vi "Monitor.vi"() -> ()   [LabVIEW 2018]
uses:
  <vilib>/Enthought/Python Integration Toolkit/api/Console Visibility.ctl
  Global Variables.vi
  <vilib>/Utility/file.llb/Read Delimited Spreadsheet (string).vi
  <vilib>/Enthought/Python Integration Toolkit/api/Unpack Bool.vi
  <vilib>/Enthought/Python Integration Toolkit/Python Integration Toolkit.lvlib
panel:
  out "Last Event Recording":string="10:59:18 AM"
  out "Sensors Info":T1(array[cluster])=[{"Label.Text"="", "Panel Ref Out"=refnum, TRUE}]
  out "Instruments":T2(array[cluster])=[{"Name"="Chassis_Sensors.vi", "vi reference"=refnum, "Running?"=TRUE}]
  in  "Add Custom Event":bool
  in  "Custom Event Str":string
  in  "Ring":u16(ring) items=["Proj_VaporTubes", "Proj_H2DT", "Proj_H2DT"]
  in  "Global File Information":T3={"Ring"=0, "SubFolder"="Temp Dependence", "Filename (Meas. Description)"="300C", "Measurement index"=5} {"Ring" items=["Proj_VaporTubes", "Proj_H2DT", "Proj_H2DT"]}
  out "File Size (Mb)":dbl[](array[numeric])
  in  "stop":bool
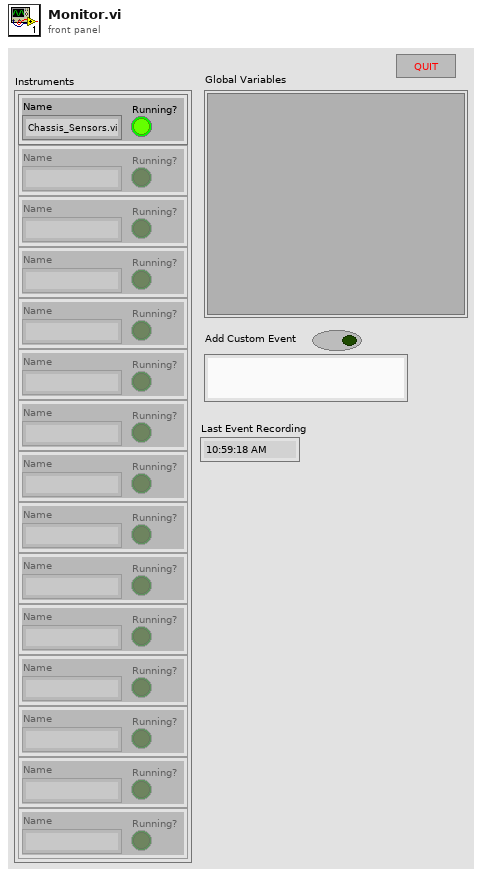
[diagram p1: front panel]
types:
  T1 = cluster{"Label.Text":string, "Panel Ref Out":refnum<vi>, bool}[]
  T2 = cluster{"Name":string, "vi reference":refnum<vi>, "Running?":bool}[]
  T3 = cluster{"Ring":u16, "SubFolder":string, "Filename (Meas. Description)":string, "Measurement index":i32}
  T4 = typedef "Python Integration Toolkit.lvlib/Console Visibility.ctl" = enum16{"Show Console", "Show Console While Running", "Hide Console"}
  T5 = enum32{"Bad", "Idle", "Run top level", "Running"}
  T6 = typedef "Python Integration Toolkit.lvlib/Session ID.ctl" = u64
  T7 = cluster{"Name":string, "vi reference":refnum<vi>, bool}
  T8 = cluster{"Name":string, "vi reference":refnum<vi>, bool}[]
  T9 = typedef "Python Integration Toolkit.lvlib/Python Objects.ctl" = variant
  T10 = cluster{"Project":u16, "SubFolder":string, "Filename (Meas. Description)":string, "Measurement index":i32}
  T11 = cluster{"Project 2":u16, "SubFolder 2":string, "Meas. Description 2":string, "Measurement number 2":i32}
  T12 = cluster{"Label.Text":bool, "Panel Ref Out":bool, bool}[]
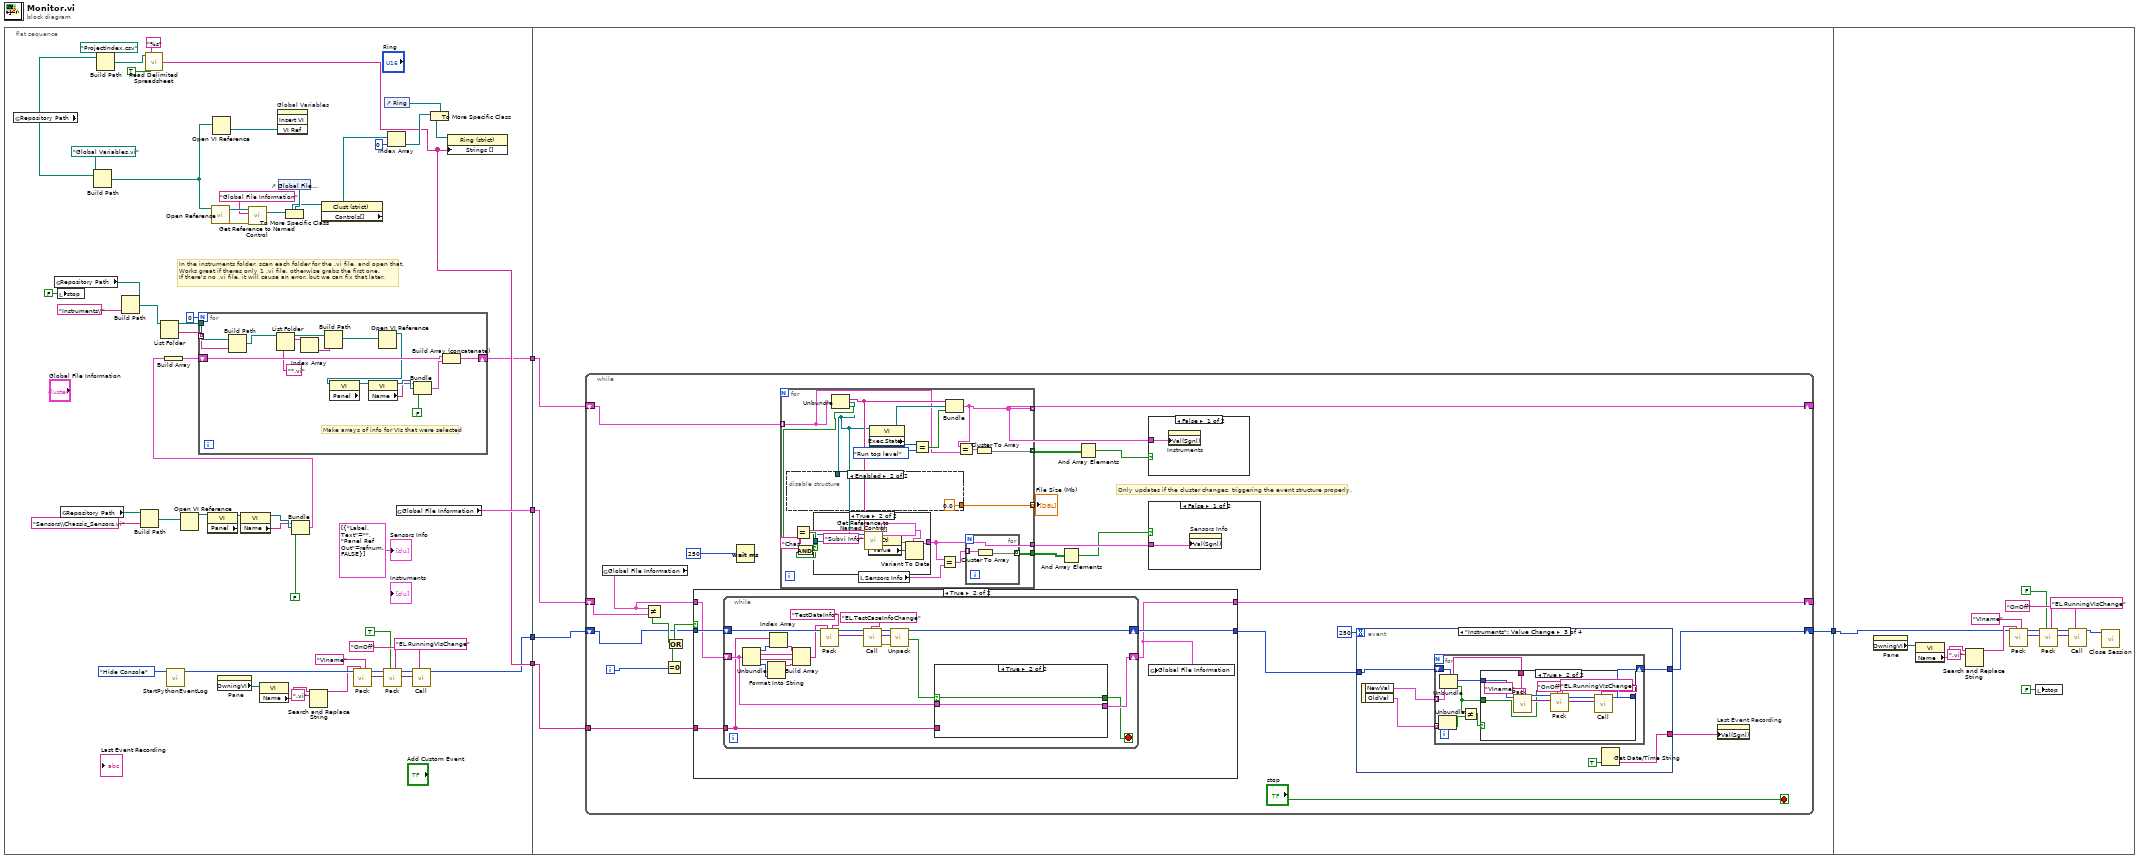
[diagram p0: block diagram]
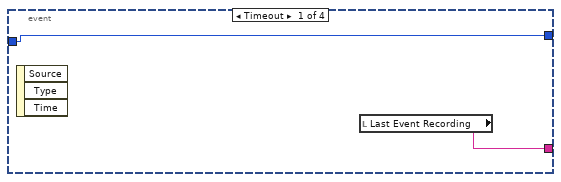
[diagram p4: hidden frame]
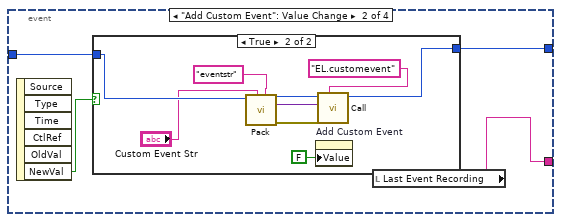
[diagram p5: hidden frame]
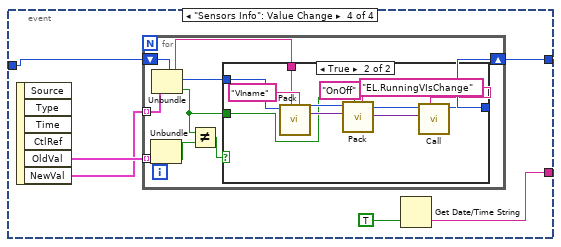
[diagram p8: hidden frame]
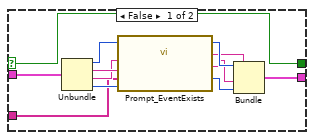
[diagram p11: hidden frame]
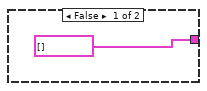
[diagram p12: hidden frame]
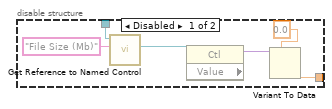
[diagram p13: hidden frame]
diagram:
  n1 = flat-sequence {
    tunnel: [w28] -> w5
    tunnel: [w41] -> w4
    tunnel: [w18] -> w2
    tunnel: [w38] -> w1
    tunnel: w5 -> [w78]
    tunnel: w4 -> [w81]
    tunnel: [w80] -> w3
    tunnel: w2 -> [w79]
    tunnel: w1 -> [w77]
    tunnel: w3 -> [w255]
    frame #0 {
      # "In the instruments folder, scan each folder for the .vi file, and open that.\nWorks great if theres only 1 .vi file, otherwise grabs the first one.\nIf there's no .vi file, it will cause an error, but we can fix that later."
      n2 = global read "Global Variables.vi" "Repository Path"() -> (w39:path)
      n3 = global read "Global Variables.vi" "Repository Path"() -> (w23:path)
      n4 = local write "stop"(FALSE ("stop")) -> ()
      n5 = global read "Global Variables.vi" "Repository Path"() -> (w17:path)
      n6 = Build Path(base path=w39, name or relative path=path "Global Variables.vi" ("vi path")) -> (appended path=w54:path)
      n7 = Build Path(base path=w39, name or relative path=path "ProjectIndex.csv" ("vi path")) -> (appended path=w42:path)
      n8 = Build Path(base path=w23, name or relative path="Instruments\\") -> (appended path=w21:path)
      n9 = Build Path(base path=w17, name or relative path="Sensors\\Chassis_Sensors.vi") -> (appended path=w15:path)
      n10 = call-poly <vilib>:"Read Delimited Spreadsheet.vi"("file path (dialog if empty)"=w42, "format (%s)"="%s", "transpose? (F)"=TRUE) -> ("first row"=w38:string[])  [unwired: 7 in, 5 out]
      n11 = List Folder(path=w21) -> (path out=w19:path, folder names=w20:string[])  [unwired: 3 in, 2 out]
      n12 = call "StartPythonEventLog.vi"("Console Visibility"=Console_Visibility."Hide Console") -> ("Session ID out"=w29:T6)  [unwired: 10 in]
      n13 = Open VI Reference(vi path=w15) -> (vi reference=w10:refnum<vi>)  [unwired: 5 in, 1 out]
      n14 = property class="VI" props=["Panel"](reference=w10) -> (reference out=w14:refnum<vi>)  [unwired: 1 in, 2 out]
      n15 = call "Open Reference.vi"("vi path"=w54) -> ("error out"=w55:errorcluster, "Front Panel Reference"=w56:refnum<vi>)  [unwired: 5 in]
      n16 = Open VI Reference(vi path=w54) -> (vi reference=w60:refnum<vi>)  [unwired: 5 in, 1 out]
      n17 = property on="Pane" class="Pane"() -> ("OwningVI"=w27:refnum<vi>)  [unwired: 2 in, 2 out]
      n18 = property class="VI"(reference=w14) -> (reference out=w13:refnum<vi>, "Name"=w11:string)  [unwired: 1 in, 1 out]
      n19 = call "Get Reference to Named Control.vi"("error in (no error)"=w55, "Control Name"="Global File Information", "Front Panel Ref"=w56) -> ("Ctl Refnum"=w52:refnum<vi>)  [unwired: 6 in, 2 out]
      n20 = property class="VI"(reference=w27) -> ("Name"=w26:string)  [unwired: 1 in, 2 out]
      n21 = invoke on="Global Variables" class="SubPnl" method="Insert VI"("VI Ref"=w60) -> ()  [unwired: 3 in, 4 out]
      n22 = control-ref of="Global File Information"() -> (w51:refnum<vi>)
      n23 = To More Specific Class(target class=w51, reference=w52) -> (specific class reference=w50:refnum<vi>)  [unwired: 1 in, 1 out]
      n24 = Bundle("Name"=w11, "vi reference"=w13, FALSE) -> (w9:T7)  [unwired: 1 in]
      n25 = Build Array(w9) -> (w8:T8)
      n26 = for {
        N: 0 -> [_]
        shift-right: [w75] -> w18
        shift-left: w8 -> [w76]
        tunnel: w19 -> [w69]
        tunnel: w20 -> [w68] mode=indexing
        # "Make arrays of info for VIs that were selected"
        n27 = Build Path(base path=w69, name or relative path=w68) -> (appended path=w63:path)
        n28 = List Folder(path=w63, pattern="*.vi") -> (path out=w62:path, filenames=w66:string[])  [unwired: 2 in, 2 out]
        n29 = Index Array(array=w66) -> (element=w65:string)  [unwired: 1 in]
        n30 = Build Path(base path=w62, name or relative path=w65) -> (appended path=w67:path)
        n31 = Open VI Reference(vi path=w67) -> (vi reference=w73:refnum<vi>)  [unwired: 5 in, 1 out]
        n32 = property class="VI" props=["Panel"](reference=w73) -> (reference out=w72:refnum<vi>)  [unwired: 1 in, 2 out]
        n33 = property class="VI"(reference=w72) -> (reference out=w71:refnum<vi>, "Name"=w61:string)  [unwired: 1 in, 1 out]
        n34 = Bundle("Name"=w61, "vi reference"=w71, FALSE) -> (w74:T7)  [unwired: 1 in]
        n35 = Build Array (concatenate)(w76, w74) -> (w75:T8)
      }
      n36 = Search and Replace String(input string=w26, search string=".vi") -> (result string=w24:string)  [unwired: 6 in, 3 out]
      n37 = property class="Clust (strict)"(reference=w50) -> ("Controls[]"=w49:refnum<vi>[])  [unwired: 1 in, 2 out]
      n38 = call <vilib>:"Pack.vi"("Keyword Name"="VIname", "Argument"=w24, "Session ID"=w29) -> ("Python Object References Out"=w33:T9, "Session ID out"=w35:T6)  [unwired: 6 in, 1 out]
      n39 = call <vilib>:"Pack.vi"("Keyword Name"="OnOff", "Argument"=TRUE, "Python Object References In"=w33, "Session ID"=w35) -> ("Python Object References Out"=w32:T9, "Session ID out"=w34:T6)  [unwired: 5 in, 1 out]
      n40 = control-ref of="Ring"() -> (w47:refnum<vi>)
      n41 = Index Array(array=w49, index=0) -> (element=w46:refnum<vi>)
      n42 = global read "Global Variables.vi" "Global File Information"() -> (w41:T10)
      n43 = call <vilib>:"Call.vi"("Function or Method Name"="EL.RunningVIsChange", "Python Object References In"=w32, "Session ID"=w34) -> ("Session ID out"=w28:T6)  [unwired: 6 in, 2 out]
      n44 = To More Specific Class(target class=w47, reference=w46) -> (specific class reference=w45:refnum<vi>)  [unwired: 1 in, 1 out]
      n45 = property class="Ring (strict)"(reference=w45, "Strings []"=w38) -> ()  [unwired: 1 in, 2 out]
      "Sensors Info" <- T1 [{"Label.Text"="", "Panel Ref Out"=refnum, FALSE}] ("Sensors Info")
    }
    frame #1 {
      n46 = while {
        shift-right: [w96] -> _
        shift-left: w81 -> [w97]
        shift-right: [w88] -> _
        shift-left: w79 -> [w87]
        shift-right: [w91] -> w80
        shift-left: w78 -> [w94]
        tunnel: w77 -> [w93]
        i -> [w100]
        stop <- "stop" stop-if-true
        # "Only updates if the cluster changes, triggering the event structure properly."
        n47 = global read "Global Variables.vi" "Global File Information"() -> (w99:T10)
        n48 = Not Equal?(x=w99, y=w97) -> (x != y?=w102:bool)
        n49 = Equal To 0?(x=w100) -> (x = 0?=w103:bool)
        n50 = Or(x=w102, y=w103) -> (x .or. y?=w98:bool)
        n51 = case shown="True" w98 {
          tunnel: w99 -> [w176 w180]
          tunnel: w94 -> [w175 w181]
          tunnel: [w176 w178] -> w96
          tunnel: [w175 w179] -> w92
          tunnel: w93 -> [_ w177]
          frame False {
          }
          frame True {
            n52 = while {
              shift-right: [w189] -> w179
              shift-left: w181 -> [w201]
              shift-right: [w186] -> w178
              shift-left: w180 -> [w187]
              tunnel: w177 -> [w184]
              stop <- w185 stop-if-true
              n53 = Unbundle(w187) -> ("Project"=w183:u16, "SubFolder"=w196:string, "Filename (Meas. Description)"=w195:string, "Measurement index"=w199:i32)
              n54 = Format Into String(w199) -> (resulting string=w194:string)  [unwired: 3 in, 1 out]
              n55 = Index Array(array=w184, index=w183) -> (element=w182:string)
              n56 = Build Array(w182, w196, w195, w194) -> (w193:string[])
              n57 = call <vilib>:"Pack.vi"("Keyword Name"="TestDataInfo", "Argument"=w193, "Session ID"=w201) -> ("Python Object References Out"=w197:T9, "Session ID out"=w198:T6)  [unwired: 6 in, 1 out]
              n58 = call <vilib>:"Call.vi"("Function or Method Name"="EL.TestCaseInfoChange", "Python Object References In"=w197, "Session ID"=w198) -> ("error out"=w192:errorcluster, "Python Object References Out"=w191:T9, "Session ID out"=w190:T6)  [unwired: 6 in]
              n59 = call-poly <vilib>:"Unpack.vi"("error in (no error)"=w192, "Python Object References In"=w191, "Session ID"=w190) -> ("Value"=w188:bool, "Session ID out"=w189:T6)  [unwired: 5 in, 2 out]
              n60 = case shown="True" w188 {
                selector: w188 -> [w204 w215]
                tunnel: w187 -> [w214 w216]
                tunnel: [w205 w216] -> w186
                tunnel: [w204 w215] -> w185
                tunnel: w184 -> [w203 _]
                frame False {
                  n61 = Unbundle(w214) -> ("Project"=w213:u16, "SubFolder"=w212:string, "Filename (Meas. Description)"=w211:string, "Measurement index"=w210:i32)
                  n62 = call "Prompt_EventExists.vi"("Project Strings"=w203, "Measurement number"=w210, "Meas. Description"=w211, "SubFolder"=w212, "Project"=w213) -> ("Meas. Description 2"=w207:string, "SubFolder 2"=w208:string, "Project 2"=w209:u16, "Measurement number 2"=w206:i32)  [unwired: 1 in]
                  n63 = Bundle("Project 2"=w209, "SubFolder 2"=w208, "Meas. Description 2"=w207, "Measurement number 2"=w206) -> (w205:T11)  [unwired: 1 in]
                }
                frame True {
                }
              }
            }
            n64 = global write "Global Variables.vi" "Global File Information"(w178) -> ()
          }
        }
        n65 = Wait (ms)(milliseconds to wait=250 ("Wait time (ms)")) -> ()  [unwired: 1 out]
        n66 = for {
          tunnel: w87 -> [w223] mode=indexing
          tunnel: [w224] -> w88 mode=indexing
          tunnel: [w233] -> w95 mode=indexing
          tunnel: [w220] -> w90
          tunnel: [w221] -> w86 mode=indexing
          tunnel: [w217] -> w83
          n67 = Unbundle(w223) -> ("Name"=w227:string, "vi reference"=w225:refnum<vi>, w229:bool)
          n68 = disable-structure shown="Enabled" {
            disable-tunnel: [w250 0.0] -> w233
            disable-tunnel: w225 -> [w249 _]
            frame Disabled {
              n69 = call "Get Reference to Named Control.vi"("Control Name"="File Size (Mb)", "Front Panel Ref"=w249) -> ("Ctl Refnum"=w247:refnum<vi>)  [unwired: 7 in, 2 out]
              n70 = property class="Ctl"(reference=w247) -> ("Value"=w252:variant)  [unwired: 1 in, 2 out]
              n71 = Variant To Data(type=0.0, Variant=w252) -> (data=w250:dbl)  [unwired: 1 in, 1 out]
            }
            frame Enabled {
            }
          }
          n72 = Equal?(x=w227, y="Chassis_Sensors.vi") -> (x = y?=w226:bool)
          n73 = And(x=w229, y=w226) -> (x .and. y?=w230:bool)
          n74 = case shown="True" w230 {
            tunnel: w225 -> [_ w246]
            tunnel: [T1 [] ("Subvi Info") w239] -> w220
            frame False {
            }
            frame True {
              n75 = call "Get Reference to Named Control.vi"("Control Name"="Subvi Info", "Front Panel Ref"=w246) -> ("error out"=w243:errorcluster, "Ctl Refnum"=w244:refnum<vi>)  [unwired: 7 in, 1 out]
              n76 = property class="Ctl"(reference=w244, error in=w243) -> (error out=w242:errorcluster, "Value"=w241:variant)  [unwired: 1 out]
              n77 = Variant To Data(error in=w242, type=T1 [] ("Subvi Info"), Variant=w241) -> (data=w239:T1)  [unwired: 1 out]
            }
          }
          n78 = local read "Sensors Info"() -> (w219:T1)
          n79 = property class="VI"(reference=w225) -> (reference out=w232:refnum<vi>, "Exec.State"=w235:T5)  [unwired: 1 in, 1 out]
          n80 = Equal?(x=w235, y=T5."Run top level" ("Execution:State 2")) -> (x = y?=w231:bool)
          n81 = Equal?(x=w220, y=w219) -> (x = y?=w218:T12)
          n82 = Bundle("Name"=w227, "vi reference"=w232, w231) -> (w224:T7)  [unwired: 1 in]
          n83 = Equal?(x=w224, y=w223) -> (x = y?=w222:cluster{"Name":bool, "vi reference":bool, bool})
          n84 = for {
            tunnel: w218 -> [w237] mode=indexing
            tunnel: [w236] -> w217 mode=indexing
            n85 = Cluster To Array(cluster=w237) -> (array=w236:bool[])
          }
          n86 = Cluster To Array(cluster=w222) -> (array=w221:bool[])
        }
        "File Size (Mb)" <- w95
        n87 = And Array Elements(Boolean array=w83) -> (logical AND=w82:bool)
        n88 = And Array Elements(Boolean array=w86) -> (logical AND=w85:bool)
        n89 = case shown="False" w85 {
          tunnel: w88 -> [w106 _]
          frame False {
            n90 = property on="Instruments" class="Arr (strict)"("Val(Sgnl)"=w106) -> ()  [unwired: 2 in, 2 out]
          }
          frame True {
          }
        }
        n91 = case shown="False" w82 {
          tunnel: w90 -> [w105 _]
          frame False {
            n92 = property on="Sensors Info" class="Arr (strict)"("Val(Sgnl)"=w105) -> ()  [unwired: 2 in, 2 out]
          }
          frame True {
          }
        }
        n93 = event shown="[2] \"Instruments\": Value Change" {
          selector: _ -> [_ _ _ _]
          dyn-events: _ -> [_ _ _ _]
          timeout: 250 -> [_ _ _ _]
          tunnel: w92 -> [w108 w111 w128 w154]
          tunnel: [w108 w110 w127 w153] -> w91
          tunnel: [w107 w109 w126 w150] -> w89
          event Timeout {
            n94 = event-data() -> ()  [unwired: 1 in, 3 out]
            n95 = local read "Last Event Recording"() -> (w107:string)
          }
          event "Add Custom Event": Value Change {
            n96 = event-data() -> ("NewVal"=w112:bool)  [unwired: 1 in, 5 out]
            n97 = case shown="True" w112 {
              tunnel: w111 -> [w113 w119]
              tunnel: [w113 w118] -> w110
              frame False {
              }
              frame True {
                n98 = call <vilib>:"Pack.vi"("Keyword Name"="eventstr", "Argument"="Custom Event Str", "Session ID"=w119) -> ("error out"=w116:errorcluster, "Python Object References Out"=w121:T9, "Session ID out"=w122:T6)  [unwired: 6 in]
                n99 = property on="Add Custom Event" class="Bool (strict)"("Value"=FALSE ("Add Custom Event")) -> ()  [unwired: 2 in, 2 out]
                n100 = call <vilib>:"Call.vi"("Function or Method Name"="EL.customevent", "error in (no error)"=w116, "Python Object References In"=w121, "Session ID"=w122) -> ("Session ID out"=w118:T6)  [unwired: 5 in, 2 out]
              }
            }
            n101 = local read "Last Event Recording"() -> (w109:string)
          }
          event "Instruments": Value Change {
            n102 = event-data() -> ("NewVal"=w124:T2, "OldVal"=w125:T2)  [unwired: 1 in]
            n103 = for {
              shift-right: [w135] -> w127
              shift-left: w128 -> [w136]
              tunnel: w124 -> [w134] mode=indexing
              tunnel: w125 -> [w132] mode=indexing
              n104 = Unbundle(w132) -> ("Running?"=w130:bool)  [unwired: 2 out]
              n105 = Unbundle(w134) -> ("Name"=w133:string, "Running?"=w129:bool)  [unwired: 1 out]
              n106 = Not Equal?(x=w129, y=w130) -> (x != y?=w131:bool)
              n107 = case shown="True" w131 {
                tunnel: w136 -> [w137 w148]
                tunnel: [w137 w146] -> w135
                tunnel: w133 -> [_ w139]
                tunnel: w129 -> [_ w138]
                frame False {
                }
                frame True {
                  n108 = call <vilib>:"Pack.vi"("Keyword Name"="VIname", "Argument"=w139, "Session ID"=w148) -> ("Python Object References Out"=w142:T9, "Session ID out"=w144:T6)  [unwired: 6 in, 1 out]
                  n109 = call <vilib>:"Pack.vi"("Keyword Name"="OnOff", "Argument"=w138, "Python Object References In"=w142, "Session ID"=w144) -> ("Python Object References Out"=w141:T9, "Session ID out"=w143:T6)  [unwired: 5 in, 1 out]
                  n110 = call <vilib>:"Call.vi"("Function or Method Name"="EL.RunningVIsChange", "Python Object References In"=w141, "Session ID"=w143) -> ("Session ID out"=w146:T6)  [unwired: 6 in, 2 out]
                }
              }
            }
            n111 = Get Date/Time String(want seconds? (F)=TRUE) -> (time string=w126:string)  [unwired: 2 in, 1 out]
          }
          event "Sensors Info": Value Change {
            n112 = event-data() -> ("OldVal"=w152:T1, "NewVal"=w151:T1)  [unwired: 1 in, 4 out]
            n113 = for {
              shift-right: [w161] -> w153
              shift-left: w154 -> [w162]
              tunnel: w151 -> [w160] mode=indexing
              tunnel: w152 -> [w158] mode=indexing
              n114 = Unbundle(w158) -> (w156:bool)  [unwired: 2 out]
              n115 = Unbundle(w160) -> ("Label.Text"=w159:string, w155:bool)  [unwired: 1 out]
              n116 = Not Equal?(x=w155, y=w156) -> (x != y?=w157:bool)
              n117 = case shown="True" w157 {
                tunnel: w162 -> [w163 w174]
                tunnel: [w163 w172] -> w161
                tunnel: w159 -> [_ w165]
                tunnel: w155 -> [_ w164]
                frame False {
                }
                frame True {
                  n118 = call <vilib>:"Pack.vi"("Keyword Name"="VIname", "Argument"=w165, "Session ID"=w174) -> ("Python Object References Out"=w168:T9, "Session ID out"=w170:T6)  [unwired: 6 in, 1 out]
                  n119 = call <vilib>:"Pack.vi"("Keyword Name"="OnOff", "Argument"=w164, "Python Object References In"=w168, "Session ID"=w170) -> ("Python Object References Out"=w167:T9, "Session ID out"=w169:T6)  [unwired: 5 in, 1 out]
                  n120 = call <vilib>:"Call.vi"("Function or Method Name"="EL.RunningVIsChange", "Python Object References In"=w167, "Session ID"=w169) -> ("Session ID out"=w172:T6)  [unwired: 6 in, 2 out]
                }
              }
            }
            n121 = Get Date/Time String(want seconds? (F)=TRUE) -> (time string=w150:string)  [unwired: 2 in, 1 out]
          }
        }
        n122 = property on="Last Event Recording" class="Str"("Val(Sgnl)"=w89) -> ()  [unwired: 2 in, 2 out]
      }
    }
    frame #2 {
      n123 = property on="Pane" class="Pane"() -> ("OwningVI"=w259:refnum<vi>)  [unwired: 2 in, 2 out]
      n124 = property class="VI"(reference=w259) -> ("Name"=w258:string)  [unwired: 1 in, 2 out]
      n125 = Search and Replace String(input string=w258, search string=".vi") -> (result string=w256:string)  [unwired: 6 in, 3 out]
      n126 = call <vilib>:"Pack.vi"("Keyword Name"="VIname", "Argument"=w256, "Session ID"=w255) -> ("Python Object References Out"=w263:T9, "Session ID out"=w265:T6)  [unwired: 6 in, 1 out]
      n127 = local write "stop"(FALSE ("stop")) -> ()
      n128 = call <vilib>:"Pack.vi"("Keyword Name"="OnOff", "Argument"=FALSE, "Python Object References In"=w263, "Session ID"=w265) -> ("Python Object References Out"=w262:T9, "Session ID out"=w264:T6)  [unwired: 5 in, 1 out]
      n129 = call <vilib>:"Call.vi"("Function or Method Name"="EL.RunningVIsChange", "Python Object References In"=w262, "Session ID"=w264) -> ("Session ID out"=w254:T6)  [unwired: 6 in, 2 out]
      n130 = call <vilib>:"Close Session.vi"("Session ID"=w254) -> ()  [unwired: 10 in, 1 out]
    }
  }
